vi "Practica4.2_ForLoop.vi"() -> ()   [LabVIEW 2022 SP3]
panel:
  out "Si  No":bool
  out "Ejecución actual":dbl(knob) scale=0.0..30.0
  in  "CantEjecuciones":dbl
  out "NumAleatorio":dbl
  in  "ValorBuscado":dbl
  # "Anahí Montserrat Vázquez Padilla \nPráctica 04: For loop \n06/02/2024"
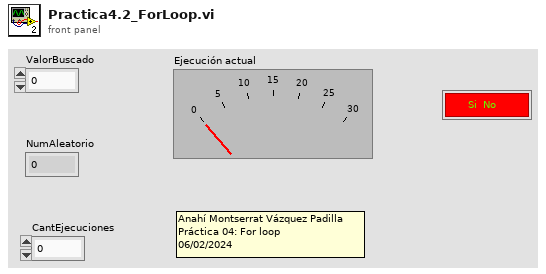
[diagram p1: front panel]
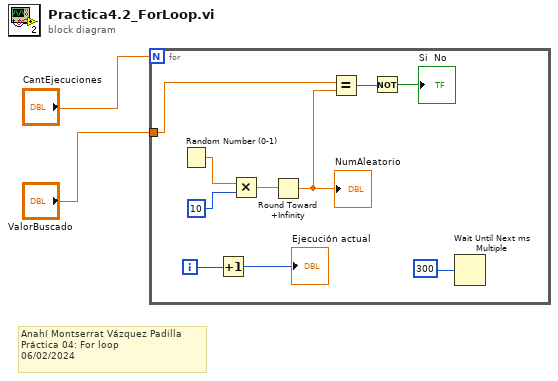
[diagram p0: block diagram]
diagram:
  # "Anahí Montserrat Vázquez Padilla \nPráctica 04: For loop \n06/02/2024"
  n1 = for {
    N: "CantEjecuciones" -> [_]
    tunnel: "ValorBuscado" -> [w7]
    i -> [w9]
    n2 = Random Number (0-1)() -> (number: 0 to 1=w11:dbl)
    n3 = Increment(x=w9) -> (x+1=→"Ejecución actual":i32)
    n4 = Multiply(x=w11, y=10) -> (x*y=w10:dbl)
    n5 = Round Toward +Infinity(x=w10) -> (ceil(x): smallest int >= x=w6:dbl)
    "NumAleatorio" <- w6
    n6 = Equal?(x=w7, y=w6) -> (x = y?=w4:bool)
    n7 = Not(x=w4) -> (.not. x?=→"Si  No":bool)
    n8 = Wait Until Next ms Multiple(millisecond multiple=300) -> ()  [unwired: 1 out]
  }
